vi "Day01-04.vi"() -> ()   [LabVIEW 2021]
panel:
  out "마지막 값":i32
  out "조건적":i32[](array[numeric])
  out "인덱스 하기":i32[](array[numeric])
  out "숫자형 3":dbl
  out "배열":dbl[](array[numeric])
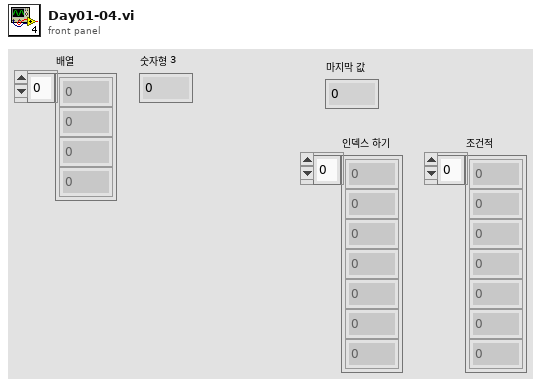
[diagram p1: front panel]
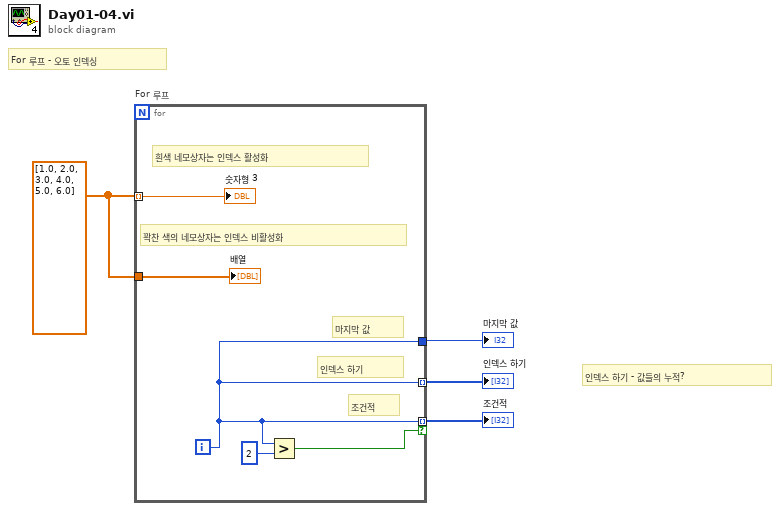
[diagram p0: block diagram]
diagram:
  w4 = dbl[] [1.0, 2.0, 3.0, 4.0, 5.0, 6.0]
  # "인덱스 하기 - 값들의 누적?"
  # "For 루프 - 오토 인덱싱"
  n1 = for "For 루프" {
    tunnel: w4 -> [w9] mode=indexing
    tunnel: w4 -> [w8]
    tunnel: [w7] -> w1
    tunnel: [w7] -> w3 mode=indexing
    tunnel: [w7] -> w2 mode=indexing if=w5
    i -> [w7]
    # "조건적"
    # "인덱스 하기"
    # "마지막 값"
    # "꽉찬 색의 네모상자는 인덱스 비활성화"
    # "흰색 네모상자는 인덱스 활성화"
    n2 = Greater?(x=w7, y=2) -> (0:w5:bool)
    "숫자형 3" <- w9
    "배열" <- w8
  }
  "인덱스 하기" <- w3
  "조건적" <- w2
  "마지막 값" <- w1
